vi "NDMotor_SetRPM.vi"() -> ()   [LabVIEW 2024]
panel:
  in  "set rpm":i32
  out "error out":errorcluster
  out "VISA resource name out":refnum<visa-resource-name>
  out "rpm":i32
  in  "error in":errorcluster
  in  "VISA resource name":refnum<visa-resource-name>
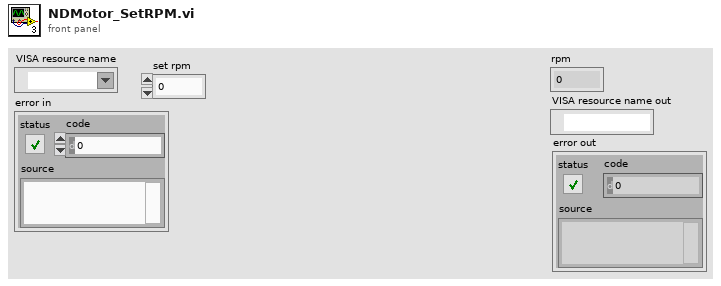
[diagram p1: front panel]
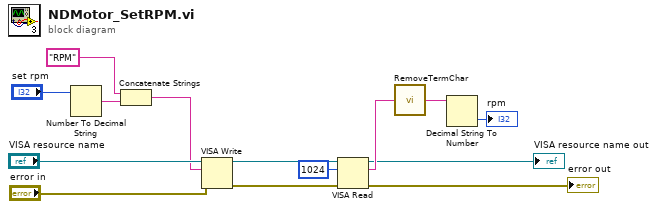
[diagram p0: block diagram]
diagram:
  n1 = Number To Decimal String(number="set rpm") -> (decimal integer string=w3:string)  [unwired: 1 in]
  n2 = Concatenate Strings("RPM" ("write buffer"), w3) -> (w1:string)
  n3 = VISA Write(VISA resource name="VISA resource name", write buffer=w1, error in (no error)="error in") -> (VISA resource name out=w11:refnum<visa-resource-name>, error out=w12:errorcluster)  [unwired: 1 out]
  n4 = VISA Read(VISA resource name=w11, byte count=u32 1024, error in (no error)=w12) -> (VISA resource name out=→"VISA resource name out":refnum<visa-resource-name>, read buffer=w9:string, error out=→"error out":errorcluster)  [unwired: 1 out]
  n5 = call "RemoveTermChar.vi"("String"=w9) -> ("Chopped String"=w8:string)  [unwired: 4 in]
  n6 = Decimal String To Number(string=w8) -> (number=→"rpm":i32)  [unwired: 2 in, 1 out]
